vi "MPS RX String.vi"(8 "error in":errorcluster, 11 "RX In":string) -> (0 "error out":errorcluster, 2 "Valid Checksum":bool, 3 "Response":string)   [LabVIEW 2025]
uses:
  <userlib>/_OpenG.lib/error/error.llb/openg_error.lvlib
panel:
  out "Checksum":u8 format="%x"
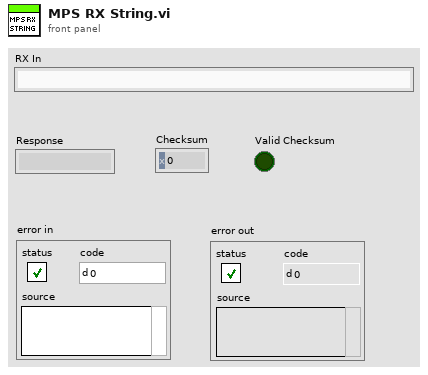
[diagram p1: front panel]
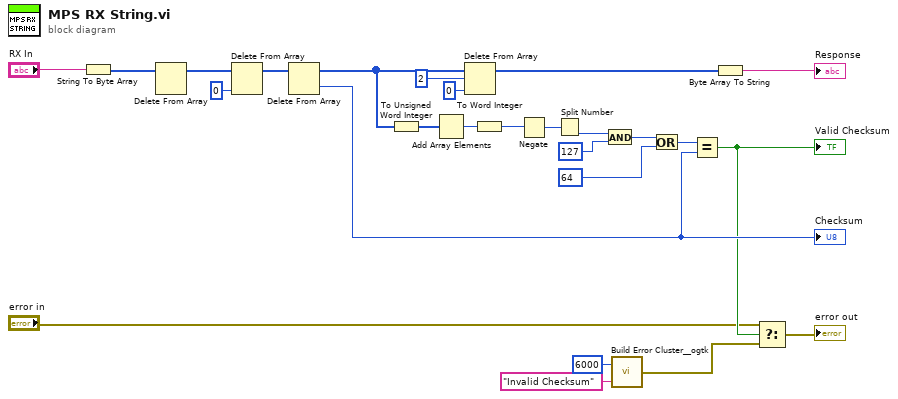
[diagram p0: block diagram]
diagram:
  n1 = String To Byte Array(string="RX In") -> (unsigned byte array=w17:u8[])
  n2 = Delete From Array(array=w17) -> (array with subset deleted=w16:u8[])  [unwired: 2 in, 1 out]
  n3 = Delete From Array(array=w16, index=0) -> (array with subset deleted=w13:u8[])  [unwired: 1 in, 1 out]
  n4 = Delete From Array(array=w13) -> (deleted portion=w11:u8, array with subset deleted=w9:u8[])  [unwired: 2 in]
  "Checksum" <- w11
  n5 = To Unsigned Word Integer(number=w9) -> (unsigned 16bit integer=w19:u16[])
  n6 = Add Array Elements(numeric array=w19) -> (sum=w20:u16)
  n7 = Delete From Array(array=w9, length=2, index=0) -> (array with subset deleted=w8:u8[])  [unwired: 1 out]
  n8 = To Word Integer(number=w20) -> (16bit integer=w21:i16)
  n9 = Negate(x=w21) -> (-x=w22:i16)
  n10 = Split Number(x=w22) -> (lo(x)=w23:u8)  [unwired: 1 out]
  n11 = And(x=w23, y=u8 127) -> (x .and. y?=w25:u8)
  n12 = call <userlib>:"Build Error Cluster__ogtk.vi"("String to Prepend to source (\"\")"="Invalid Checksum" ("String to Prepend to source (\"\")"), "code"=6000) -> ("error out"=w1:errorcluster)
  n13 = Or(x=w25, y=u8 64) -> (x .or. y?=w12:u8)
  n14 = Equal?(x=w12, y=w11) -> (x = y?=w6:bool)
  "Valid Checksum" <- w6
  n15 = Byte Array To String(unsigned byte array=w8) -> (string=→"Response":string)
  n16 = Select(t="error in", s=w6, f=w1) -> (s? t:f=→"error out":errorcluster)
